vi "GetLocalAddress.vi"(11 "Error In":errorcluster) -> (4 "IP Address":string, 15 "Error Out":errorcluster)   [LabVIEW 2020]
uses:
  <vilib>/Utility/error.llb/whitespace.ctl
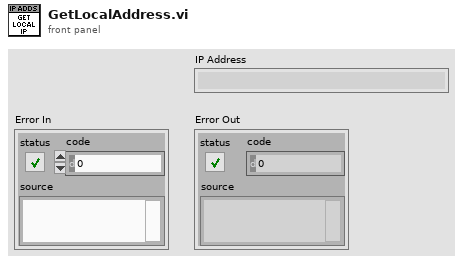
[diagram p1: front panel]
types:
  T1 = typedef "whitespace.ctl" = u16
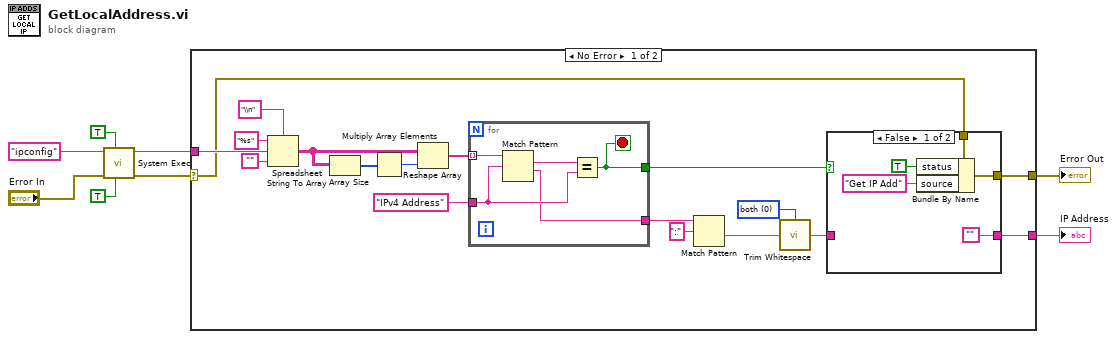
[diagram p0: block diagram]
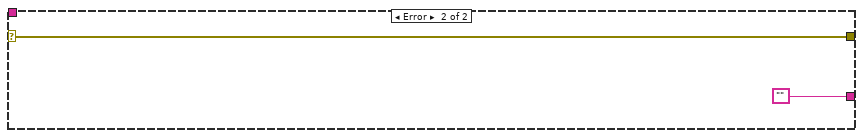
[diagram p3: hidden frame]
diagram:
  n1 = call <vilib>:"System Exec.vi"("run minimized? (F)"=TRUE, "wait until completion? (T)"=TRUE, "error in (no error)"="Error In", "command line"="ipconfig") -> ("error out"=w4:errorcluster, "standard output"=w5:string)  [unwired: 4 in, 2 out]
  n2 = case shown="No Error" w4 {
    selector: w4 -> [w11 w39]
    tunnel: w5 -> [w26 _]
    tunnel: [w10 ""] -> w3
    tunnel: [w9 w39] -> w1
    frame No Error {
      w14 = T1 0 items=["both", "start of string", "end of string"] ("location (both)")
      n3 = Spreadsheet String To Array(delimiter (Tab)="\\n", format string="%s", spreadsheet string=w26, array type (2D Dbl)="") -> (array=w21:string[][])
      n4 = Array Size(array=w21) -> (size(s)=w22:i32[])
      n5 = Multiply Array Elements(1:w22) -> (0:w20:i32)
      n6 = Reshape Array(w21, w20) -> (w19:string[])
      n7 = for {
        tunnel: w19 -> [w38] mode=indexing
        tunnel: "IPv4 Address" ("command line") -> [w36]
        tunnel: [w35] -> w17
        tunnel: [w34] -> w13
        stop <- w34 stop-if-true
        n8 = Match Pattern(string=w38, regular expression=w36) -> (match substring=w37:string, after substring=w35:string)  [unwired: 1 in, 2 out]
        n9 = Equal?(x=w37, y=w36) -> (x = y?=w34:bool)
      }
      n10 = Match Pattern(string=w17, regular expression=":") -> (after substring=w15:string)  [unwired: 1 in, 3 out]
      n11 = call <vilib>:"Trim Whitespace.vi"("string"=w15, "location (both)"=w14) -> ("trimmed string"=w12:string)
      n12 = case shown="False" w13 {
        tunnel: w12 -> [_ w33]
        tunnel: w11 -> [w30 w32]
        tunnel: ["" w33] -> w10
        tunnel: [w27 w32] -> w9
        frame False {
          n13 = Bundle By Name(cluster=w30, "status"=TRUE, "source"="Get IP Add") -> (w27:errorcluster)
        }
        frame True {
        }
      }
    }
    frame Error {
    }
  }
  "IP Address" <- w3
  "Error Out" <- w1
